vi "myRIO_BRIG_RT__testFPGA_time.vi"() -> ()   [LabVIEW 2014]
uses:
  <vilib>/myRIO/Common/Instrument Driver Framework/myRIO v1.0/UART/vis/myRIO v1.0 Close UART.vi
  <vilib>/FPGAPlugInAG/myRIO-1900/niLvFpga_Open_myRIO-1900.vi
  <vilib>/rvi/interface/common/dynamic/niFpgaDynamicAddResources.vi
  <vilib>/Utility/error.llb/Error Cluster From Error Code.vi
  <vilib>/rvi/errors/niLvFpgaAdjustHostInterfaceError.vi
  <vilib>/FPGAPlugInAG/Dynamic/niLvFpga_Close_Dynamic.vi
  <vilib>/myRIO/Common/Instrument Driver Framework/Utilities/vis/FPGA Ref Manager.vi
  <vilib>/myRIO/Common/Instrument Driver Framework/myRIO v1.0/myRIO v1.0 Reset FPGA.vi
  <vilib>/myRIO/Common/Instrument Driver Framework/myRIO v1.0/IRQ/vis/myRIO v1.0 IRQ Info FGV.vi
  <vilib>/myRIO/Common/Instrument Driver Framework/myRIO v1.0/IRQ/vis/myRIO v1.0 Timer IRQ Info FGV.vi
  <vilib>/myRIO/Common/Instrument Driver Framework/myRIO v1.0/IRQ/vis/myRIO v1.0 ISR Agent.vi
  <vilib>/rvi/interface/nirviOpenFPGA/nirviOpenFPGA.xnode
  FPGA Bitfiles/myRIOBRig_FPGATarget_myRIOBRigFPGAv3,_rBLkV1r30v0.lvbitx
  myRIO_BRig_FPGA_v3,51__PortC__testSinwave.vi
  <vilib>/rvi/interface/nirviReadWriteControl/nirviReadWriteControl.xnode
  <vilib>/rvi/interface/nirviCloseFPGA/nirviCloseFPGA.xnode
  NiFpgaLv.dll
  <vilib>/rvi/interface/Simulation/niFpgaSimulationCallBeginRW.vi
  <vilib>/myRIO/Instrument Drivers/Utilities/Utilities.lvlib
panel:
  in  "stop":bool
  out "k1_counts/ms":dbl
  in  "time [ms]":u16=60000
  in  "timeTrial":bool
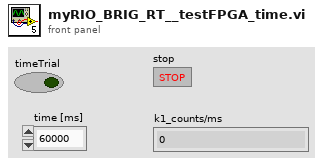
[diagram p1: front panel]
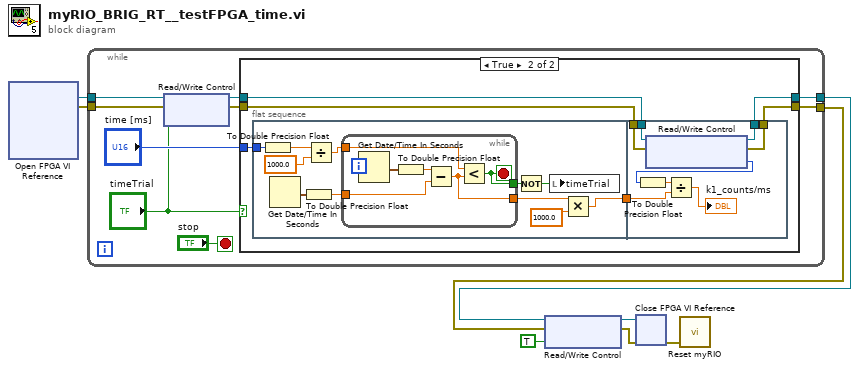
[diagram p0: block diagram]
diagram:
  n1 = xnode "Open FPGA VI Reference"() -> ("FPGA VI Reference Out"=w8:refnum<k20>, "error out"=w7:errorcluster)  [unwired: 2 in]
  n2 = while {
    tunnel: w8 -> [w16]
    tunnel: w7 -> [w15]
    tunnel: [w11] -> w1
    tunnel: [w10] -> w2
    stop <- "stop" stop-if-true
    n3 = xnode "Read/Write Control"("FPGA VI Reference In"=w16, "error in"=w15, "timeTrial"="timeTrial") -> ("FPGA VI Reference Out"=w13:refnum<k20>, "error out"=w12:errorcluster)
    n4 = case shown="True" "timeTrial" {
      tunnel: "time [ms]" -> [_ w25]
      tunnel: w13 -> [w19 w24]
      tunnel: w12 -> [w18 w23]
      tunnel: [w19 w21] -> w11
      tunnel: [w18 w20] -> w10
      frame False {
      }
      frame True {
        n5 = flat-sequence {
          tunnel: w25 -> [w34]
          tunnel: [w26] -> w22
          tunnel: w24 -> [w50]
          tunnel: w23 -> [w49]
          tunnel: w22 -> [w46]
          tunnel: [w44] -> w21
          tunnel: [w43] -> w20
          frame #0 {
            n6 = To Double Precision Float(number=w34) -> (double precision float=w31:dbl)
            n7 = Get Date/Time In Seconds() -> (seconds since 1Jan1904=w36:timestamp)
            n8 = To Double Precision Float(number=w36) -> (double precision float=w35:dbl)
            n9 = Divide(x=w31, y=1000.0) -> (x/y=w30:dbl)
            n10 = while {
              tunnel: w35 -> [w40]
              tunnel: w30 -> [w38]
              tunnel: [w39] -> w33
              tunnel: [w37] -> w27
              stop <- w39 stop-if-true
              n11 = Get Date/Time In Seconds() -> (seconds since 1Jan1904=w42:timestamp)
              n12 = To Double Precision Float(number=w42) -> (double precision float=w41:dbl)
              n13 = Subtract(x=w41, y=w40) -> (x-y=w37:dbl)
              n14 = Less?(x=w38, y=w37) -> (x < y?=w39:bool)
            }
            n15 = Not(x=w33) -> (.not. x?=w32:bool)
            n16 = local write "timeTrial"(w32) -> ()
            n17 = Multiply(x=w27, y=1000.0) -> (x*y=w26:dbl)
          }
          frame #1 {
            n18 = xnode "Read/Write Control"("FPGA VI Reference In"=w50, "error in"=w49) -> ("FPGA VI Reference Out"=w44:refnum<k20>, "error out"=w43:errorcluster, "count_timeTrial"=w48:u32)
            n19 = To Double Precision Float(number=w48) -> (double precision float=w47:dbl)
            n20 = Divide(x=w47, y=w46) -> (x/y=→"k1_counts/ms":dbl)
          }
        }
      }
    }
  }
  n21 = xnode "Read/Write Control"("FPGA VI Reference In"=w1, "error in"=w2, "FPGA_Stop"=TRUE) -> ("FPGA VI Reference Out"=w4:refnum<k20>, "error out"=w5:errorcluster)
  n22 = xnode "Close FPGA VI Reference"("FPGA VI Reference In"=w4, "error in"=w5) -> ("error out"=w3:errorcluster)
  n23 = call <vilib>:"Reset myRIO.vi"("error in (no error)"=w3) -> ()  [unwired: 10 in, 1 out]
